vi "a..a构成的数列之和.vi"(11 "a":i32=100) -> (3 "Sn":i32)   [LabVIEW 2012]
doc: "功能：\n\n求自然数的平方和。\n\n公式：\n\nSn=1^2+2^....+n^2\n\ncsxcs_366创建"
panel:
  in  "n":i32=100
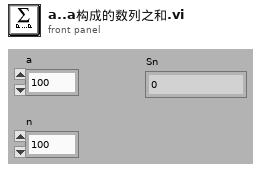
[diagram p1: front panel]
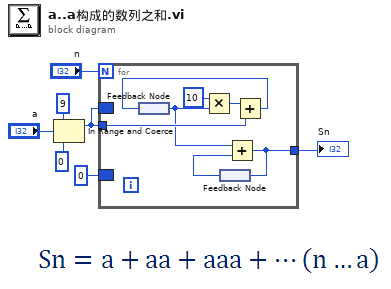
[diagram p0: block diagram]
diagram:
  n1 = In Range and Coerce(upper limit=9 ("上限"), x="a", lower limit=0 ("下限")) -> (coerced(x)=w1:i32)  [unwired: 1 out]
  n2 = for {
    N: "n" -> [_]
    tunnel: w1 -> [w11]
    tunnel: [w8] -> w3
    border: 0 ("下限") -> [_]
    border: w1 -> [_]
    n3 = feedback #1() -> (w10:i32)
    n4 = Multiply(x=10 ("y"), y=w10) -> (x*y=w13:i32)
    n5 = feedback #2() -> (w9:i32)
    n6 = Add(x=w10, y=w9) -> (x+y=w8:i32)
    n7 = feedback-in #2(w8) -> ()
    n8 = Add(x=w13, y=w11) -> (x+y=w12:i32)
    n9 = feedback-in #1(w12) -> ()
  }
  "Sn" <- w3
